vi "Flatten Type.vi"(8 "error in (no error)":errorcluster, 11 "Stream in":refnum<class "Stream.lvclass">) -> (0 "error out":errorcluster, 2 "Flatten Type":T1, 3 "Stream out":refnum<class "Stream.lvclass">)   [LabVIEW 2020, in "Stream.lvlib" / "Stream.lvclass"]
uses:
  Stream.lvclass
  Flatten Type.ctl
  Stream.lvlib
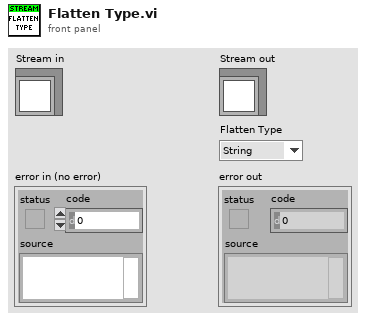
[diagram p1: front panel]
types:
  T1 = typedef "Stream.lvlib/Flatten Type.ctl" = enum16{"String", "JSON", "Custom"}
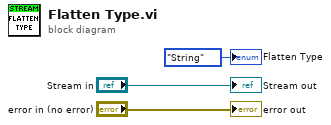
[diagram p0: block diagram]
diagram:
  "error out" <- "error in (no error)"
  "Stream out" <- "Stream in"
  "Flatten Type" <- Flatten_Type."String" ("Flatten Type")
